vi "UTEX Write Check Valid.vi"(8 "error in":errorcluster, 10 "write buffer":string="PW7", 11 "VISA Refnum in":refnum<visa-resource-name>="COM4") -> (0 "error out":errorcluster, 1 "Good Command?":bool, 2 "read buffer":string, 3 "VISA Refnum out":refnum<visa-resource-name>)   [LabVIEW 2022 SP3]
panel:
  out "match substring":string
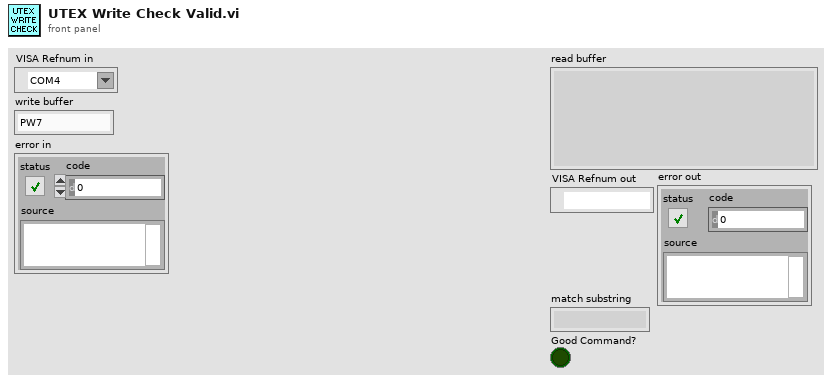
[diagram p1: front panel]
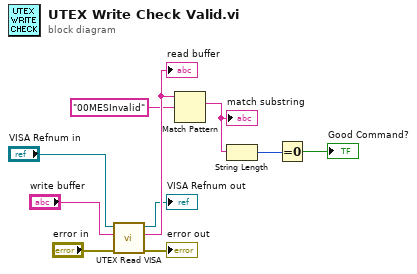
[diagram p0: block diagram]
diagram:
  n1 = call "UTEX Read VISA.vi"("error in"="error in", "write buffer"="write buffer", "VISA Refnum in"="VISA Refnum in") -> ("error out"=→"error out":errorcluster, "read buffer"=w8:string, "VISA Refnum out"=→"VISA Refnum out":refnum<visa-resource-name>)  [unwired: 6 in]
  "read buffer" <- w8
  n2 = Match Pattern(string=w8, regular expression="00MESInvalid") -> (match substring=w6:string)  [unwired: 1 in, 3 out]
  "match substring" <- w6
  n3 = String Length(string=w6) -> (length=w5:i32)
  n4 = Equal To 0?(x=w5) -> (x = 0?=→"Good Command?":bool)
